vi "Scale.vi"(8 "error in (no error)":errorcluster, 10 "Scale Factor":dbl, 11 "Circle in":refnum<class "Circle.lvclass">) -> (0 "error out":errorcluster, 3 "Circle out":refnum<class "Circle.lvclass">)   [LabVIEW 2021, in "Picture2D.lvlib" / "Circle.lvclass"]
uses:
  Circle.lvclass
  Circle.lvclass/Circle.ctl
  Shape/Shape.lvclass
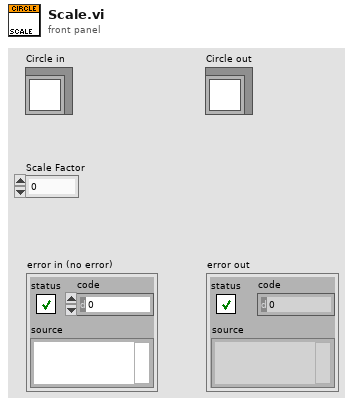
[diagram p1: front panel]
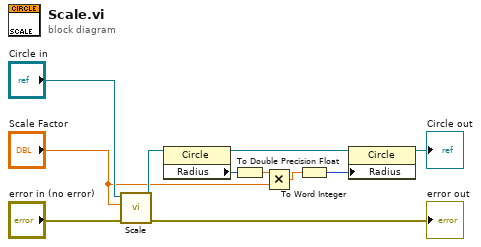
[diagram p0: block diagram]
diagram:
  n1 = call-parent "Scale.vi"("error in (no error)"="error in (no error)", "Scale Factor"="Scale Factor", "Shape in"="Circle in") -> ("error out"=→"error out":errorcluster, "Shape out"=w10:refnum<class "Circle.lvclass">)  [unwired: 7 in]
  n2 = property class="Circle"(reference=w10) -> (reference out=w7:refnum<class "Circle.lvclass">, "Radius"=w5:i16)  [unwired: 1 in, 1 out]
  n3 = To Double Precision Float(number=w5) -> (double precision float=w1:dbl)
  n4 = Multiply(x=w1, y="Scale Factor") -> (x*y=w3:dbl)
  n5 = To Word Integer(number=w3) -> (16bit integer=w2:i16)
  n6 = property class="Circle"(reference=w7, "Radius"=w2) -> (reference out=→"Circle out":refnum<class "Circle.lvclass">)  [unwired: 1 in, 1 out]
